vi "View-Scheme.vi"(11 "Material-Scheme.lvclass":refnum<class "Material-Scheme.lvclass">) -> ()   [LabVIEW 2021, in "TSC Material Theme.lvlib" / "Material-Scheme.lvclass"]
doc: "scheme view UI set up like the material theme display\n\n<b>Code Developed By:</b>\nTechnology Service Corporation\nwww.tsc.com/atcs\n\nDeveloper:\nDaniel Coons"
uses:
  Material-Scheme.lvclass
  <vilib>/Utility/traverseref.llb/TRef TravTarget.ctl
  Material-Scheme.lvclass/Material-Scheme.ctl
  <vilib>/Utility/colorconv.llb/Color to RGB.vi
  <vilib>/Utility/traverseref.llb/VI Scripting - Traverse.lvlib
panel:
  out "Scrim":u32(colorbox)
  out "Shadow":u32(colorbox)
  out "Inverse Primary":u32(colorbox)
  out "Inverse on Surface":u32(colorbox)
  out "Inverse Surface":u32(colorbox)
  out "On Error Container":u32(colorbox)
  out "Error Container":u32(colorbox)
  out "On Error":u32(colorbox)
  out "Error":u32(colorbox)
  out "Outline":u32(colorbox)
  out "Outline Variant":u32(colorbox)
  out "On Surface Var":u32(colorbox)
  out "On Surface":u32(colorbox)
  out "Surf Container Highest":u32(colorbox)
  out "Surf Container":u32(colorbox)
  out "Surf Container High":u32(colorbox)
  out "Surf Container Low":u32(colorbox)
  out "Surf Container Lowest":u32(colorbox)
  out "Surface Bright":u32(colorbox)
  out "Surface":u32(colorbox)
  out "Surface Dim":u32(colorbox)
  out "Tertiary Fixed":u32(colorbox)
  out "On Tertiary Fixed Variant":u32(colorbox)
  out "On Tertiary Fixed":u32(colorbox)
  out "Tertiary Fixed Dim":u32(colorbox)
  out "On Tertiary Container":u32(colorbox)
  out "Tertiary Container":u32(colorbox)
  out "On Tertiary":u32(colorbox)
  out "Tertiary":u32(colorbox)
  out "Secondary Fixed":u32(colorbox)
  out "On Secondary Fixed Variant":u32(colorbox)
  out "On Secondary Fixed":u32(colorbox)
  out "Secondary Fixed Dim":u32(colorbox)
  out "On Secondary Container":u32(colorbox)
  out "Secondary Container":u32(colorbox)
  out "On Secondary":u32(colorbox)
  out "Secondary":u32(colorbox)
  out "On Primary Fixed Variant":u32(colorbox)
  out "On Primary Fixed":u32(colorbox)
  out "Primary Fixed Dim":u32(colorbox)
  out "Primary Fixed":u32(colorbox)
  out "On Primary Container":u32(colorbox)
  out "Primary Container":u32(colorbox)
  out "On Primary":u32(colorbox)
  out "Primary":u32(colorbox)
  # "Hover to see color pattern and click to change..."
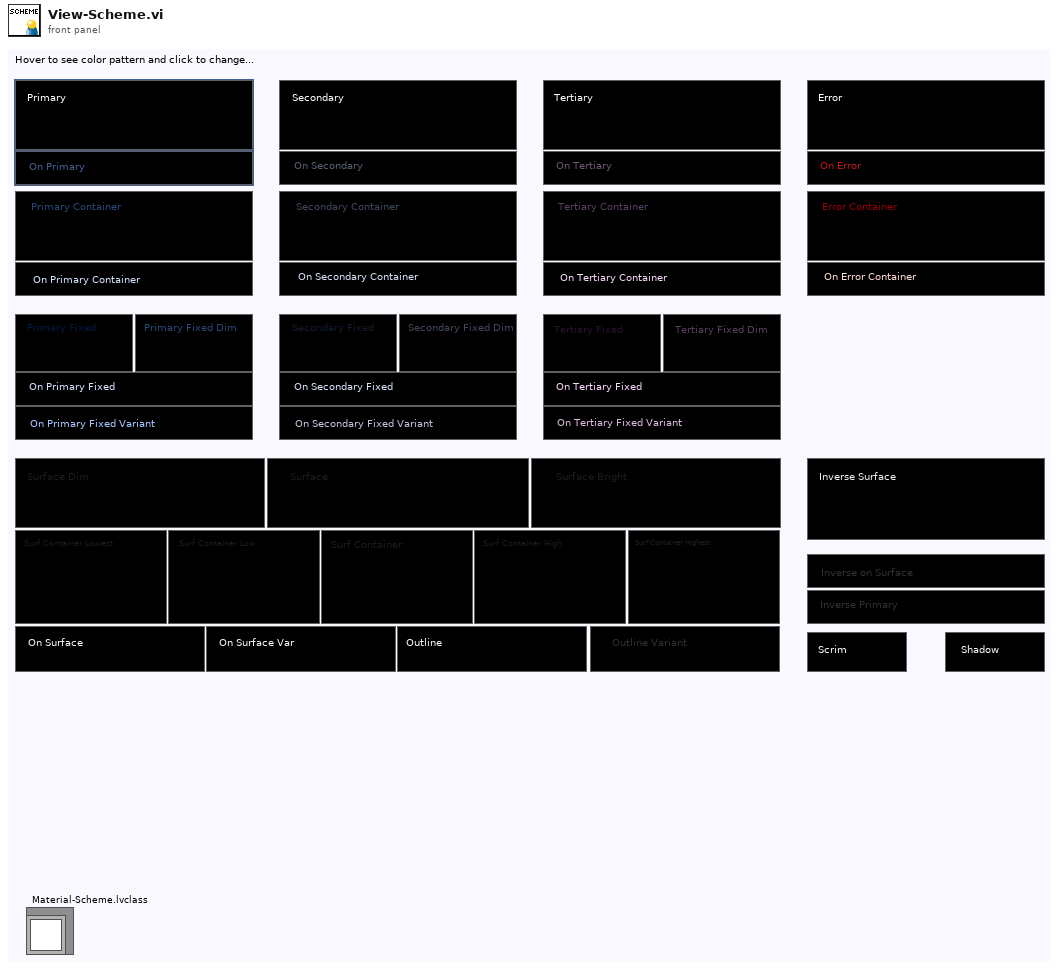
[diagram p1: front panel]
types:
  T1 = typedef "TRef TravTarget.ctl" = enum16{"FP", "BD", "Other"}
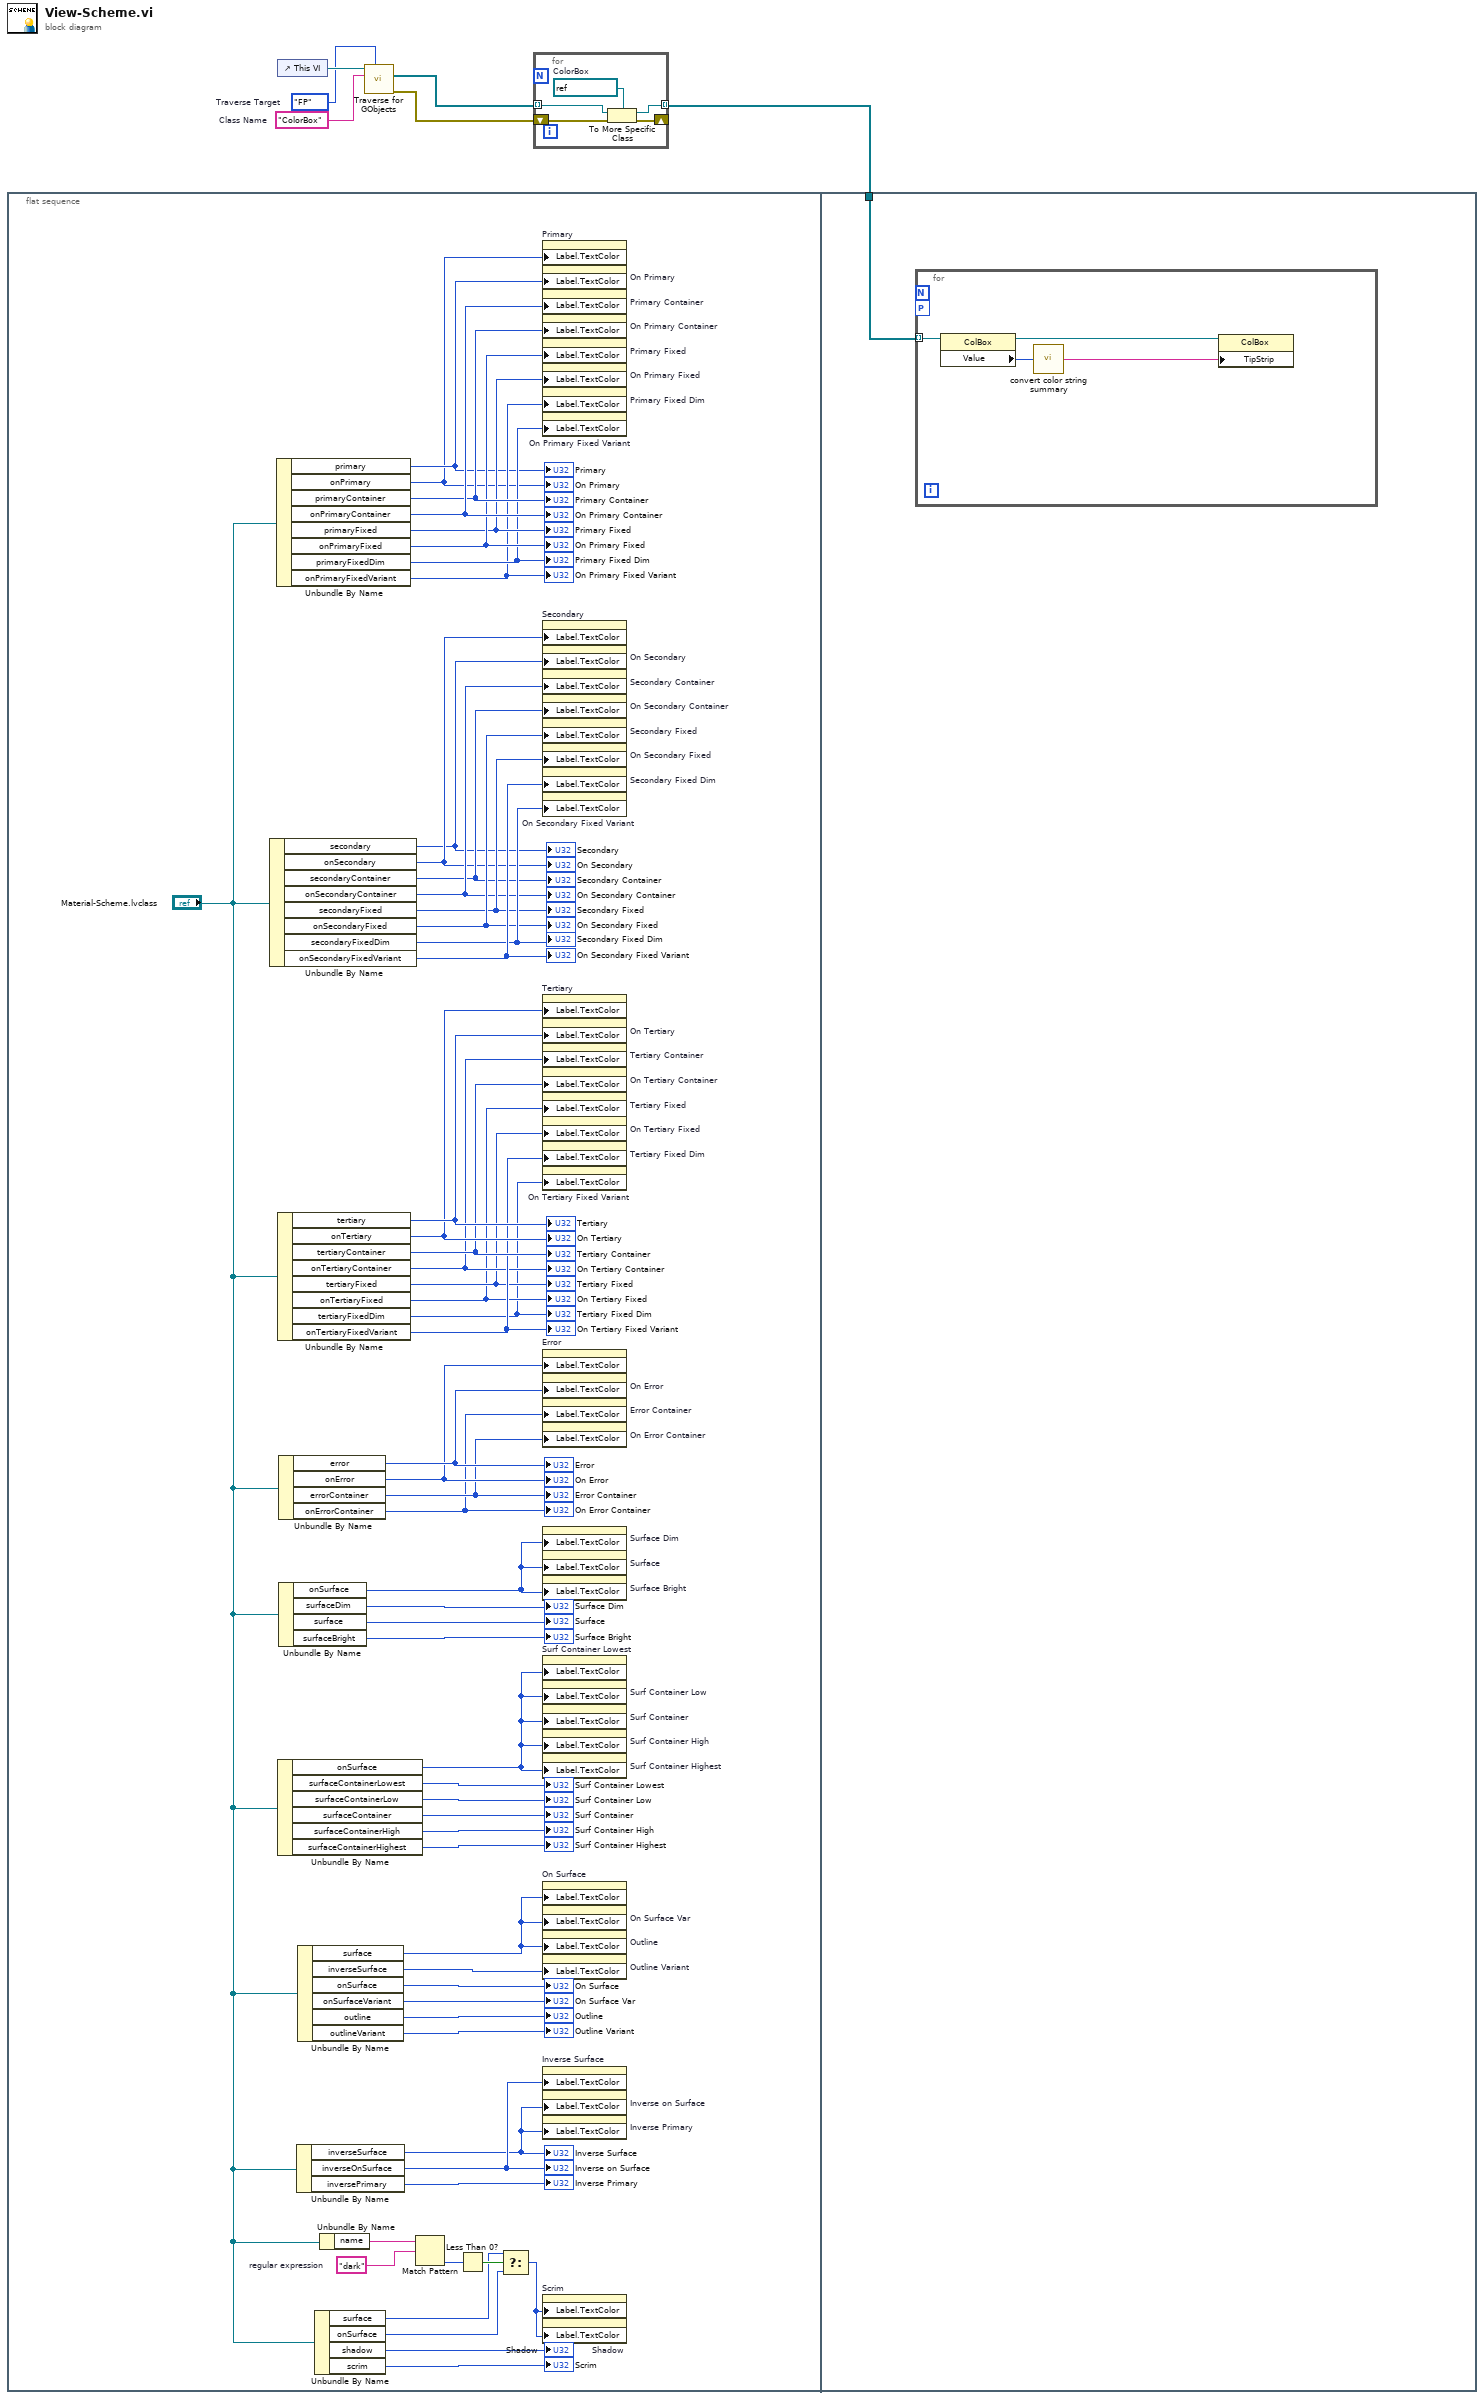
[diagram p0: block diagram]
diagram:
  w3 = TRef_TravTarget."FP"  # Traverse Target
  w6 = "ColorBox"  # Class Name
  n1 = flat-sequence {
    tunnel: w1 -> [w64]
    frame #0 {
      w14 = "dark"  # regular expression
      n2 = Unbundle By Name("Material-Scheme.lvclass") -> ("secondary"=w50:u32, "onSecondary"=w51:u32, "secondaryContainer"=w52:u32, "onSecondaryContainer"=w53:u32, "secondaryFixed"=w54:u32, "onSecondaryFixed"=w55:u32, "secondaryFixedDim"=w56:u32, "onSecondaryFixedVariant"=w57:u32)
      "Secondary" <- w50
      "On Secondary" <- w51
      "Secondary Container" <- w52
      "On Secondary Container" <- w53
      "Secondary Fixed Dim" <- w56
      "On Secondary Fixed" <- w55
      "On Secondary Fixed Variant" <- w57
      "Secondary Fixed" <- w54
      n3 = Unbundle By Name("Material-Scheme.lvclass") -> ("primary"=w8:u32, "onPrimary"=w7:u32, "primaryContainer"=w62:u32, "onPrimaryContainer"=w63:u32, "primaryFixed"=w60:u32, "onPrimaryFixed"=w61:u32, "primaryFixedDim"=w59:u32, "onPrimaryFixedVariant"=w58:u32)
      "Primary" <- w8
      "On Primary" <- w7
      "Primary Container" <- w62
      "On Primary Container" <- w63
      "Primary Fixed" <- w60
      "Primary Fixed Dim" <- w59
      "On Primary Fixed" <- w61
      "On Primary Fixed Variant" <- w58
      n4 = Unbundle By Name("Material-Scheme.lvclass") -> ("tertiary"=w49:u32, "onTertiary"=w48:u32, "tertiaryContainer"=w47:u32, "onTertiaryContainer"=w45:u32, "tertiaryFixed"=w44:u32, "onTertiaryFixed"=w43:u32, "tertiaryFixedDim"=w42:u32, "onTertiaryFixedVariant"=w46:u32)
      "Tertiary" <- w49
      "On Tertiary" <- w48
      "Tertiary Container" <- w47
      "On Tertiary Container" <- w45
      "Tertiary Fixed Dim" <- w42
      "On Tertiary Fixed" <- w43
      "On Tertiary Fixed Variant" <- w46
      "Tertiary Fixed" <- w44
      n5 = Unbundle By Name("Material-Scheme.lvclass") -> ("onSurface"=w28:u32, "surfaceContainerLowest"=→"Surf Container Lowest":u32, "surfaceContainerLow"=→"Surf Container Low":u32, "surfaceContainer"=→"Surf Container":u32, "surfaceContainerHigh"=→"Surf Container High":u32, "surfaceContainerHighest"=→"Surf Container Highest":u32)
      n6 = Unbundle By Name("Material-Scheme.lvclass") -> ("error"=w41:u32, "onError"=w40:u32, "errorContainer"=w39:u32, "onErrorContainer"=w38:u32)
      "Error" <- w41
      "On Error" <- w40
      "Error Container" <- w39
      "On Error Container" <- w38
      n7 = Unbundle By Name("Material-Scheme.lvclass") -> ("onSurface"=w34:u32, "surfaceDim"=→"Surface Dim":u32, "surface"=→"Surface":u32, "surfaceBright"=→"Surface Bright":u32)
      n8 = Unbundle By Name("Material-Scheme.lvclass") -> ("inverseSurface"=w19:u32, "inverseOnSurface"=w20:u32, "inversePrimary"=→"Inverse Primary":u32)
      "Inverse Surface" <- w19
      "Inverse on Surface" <- w20
      n9 = Unbundle By Name("Material-Scheme.lvclass") -> ("surface"=w23:u32, "inverseSurface"=w22:u32, "onSurface"=→"On Surface":u32, "onSurfaceVariant"=→"On Surface Var":u32, "outline"=→"Outline":u32, "outlineVariant"=→"Outline Variant":u32)
      n10 = Unbundle By Name("Material-Scheme.lvclass") -> ("surface"=w11:u32, "onSurface"=w10:u32, "shadow"=→"Shadow":u32, "scrim"=→"Scrim":u32)
      n11 = Unbundle By Name("Material-Scheme.lvclass") -> ("name"=w15:string)
      n12 = Match Pattern(string=w15, regular expression=w14) -> (offset past match=w13:i32)  [unwired: 1 in, 3 out]
      n13 = Less Than 0?(x=w13) -> (x < 0?=w12:bool)
      n14 = Select(t=w11, s=w12, f=w10) -> (s? t:f=w9:u32)
      n15 = property on="Primary" class="ColBox"("Label.TextColor"=w7) -> ()  [unwired: 2 in, 2 out]
      n16 = property on="On Primary" class="ColBox"("Label.TextColor"=w8) -> ()  [unwired: 2 in, 2 out]
      n17 = property on="Primary Container" class="ColBox"("Label.TextColor"=w63) -> ()  [unwired: 2 in, 2 out]
      n18 = property on="On Primary Container" class="ColBox"("Label.TextColor"=w62) -> ()  [unwired: 2 in, 2 out]
      n19 = property on="Primary Fixed" class="ColBox"("Label.TextColor"=w61) -> ()  [unwired: 2 in, 2 out]
      n20 = property on="On Primary Fixed" class="ColBox"("Label.TextColor"=w60) -> ()  [unwired: 2 in, 2 out]
      n21 = property on="Primary Fixed Dim" class="ColBox"("Label.TextColor"=w58) -> ()  [unwired: 2 in, 2 out]
      n22 = property on="On Primary Fixed Variant" class="ColBox"("Label.TextColor"=w59) -> ()  [unwired: 2 in, 2 out]
      n23 = property on="Secondary" class="ColBox"("Label.TextColor"=w51) -> ()  [unwired: 2 in, 2 out]
      n24 = property on="On Secondary" class="ColBox"("Label.TextColor"=w50) -> ()  [unwired: 2 in, 2 out]
      n25 = property on="Secondary Container" class="ColBox"("Label.TextColor"=w53) -> ()  [unwired: 2 in, 2 out]
      n26 = property on="On Secondary Container" class="ColBox"("Label.TextColor"=w52) -> ()  [unwired: 2 in, 2 out]
      n27 = property on="Secondary Fixed" class="ColBox"("Label.TextColor"=w55) -> ()  [unwired: 2 in, 2 out]
      n28 = property on="On Secondary Fixed" class="ColBox"("Label.TextColor"=w54) -> ()  [unwired: 2 in, 2 out]
      n29 = property on="Secondary Fixed Dim" class="ColBox"("Label.TextColor"=w57) -> ()  [unwired: 2 in, 2 out]
      n30 = property on="On Secondary Fixed Variant" class="ColBox"("Label.TextColor"=w56) -> ()  [unwired: 2 in, 2 out]
      n31 = property on="Tertiary" class="ColBox"("Label.TextColor"=w48) -> ()  [unwired: 2 in, 2 out]
      n32 = property on="On Tertiary" class="ColBox"("Label.TextColor"=w49) -> ()  [unwired: 2 in, 2 out]
      n33 = property on="Tertiary Container" class="ColBox"("Label.TextColor"=w45) -> ()  [unwired: 2 in, 2 out]
      n34 = property on="On Tertiary Container" class="ColBox"("Label.TextColor"=w47) -> ()  [unwired: 2 in, 2 out]
      n35 = property on="Tertiary Fixed" class="ColBox"("Label.TextColor"=w43) -> ()  [unwired: 2 in, 2 out]
      n36 = property on="On Tertiary Fixed" class="ColBox"("Label.TextColor"=w44) -> ()  [unwired: 2 in, 2 out]
      n37 = property on="Tertiary Fixed Dim" class="ColBox"("Label.TextColor"=w46) -> ()  [unwired: 2 in, 2 out]
      n38 = property on="On Tertiary Fixed Variant" class="ColBox"("Label.TextColor"=w42) -> ()  [unwired: 2 in, 2 out]
      n39 = property on="Error" class="ColBox"("Label.TextColor"=w40) -> ()  [unwired: 2 in, 2 out]
      n40 = property on="On Error" class="ColBox"("Label.TextColor"=w41) -> ()  [unwired: 2 in, 2 out]
      n41 = property on="Error Container" class="ColBox"("Label.TextColor"=w38) -> ()  [unwired: 2 in, 2 out]
      n42 = property on="On Error Container" class="ColBox"("Label.TextColor"=w39) -> ()  [unwired: 2 in, 2 out]
      n43 = property on="Surface Dim" class="ColBox"("Label.TextColor"=w34) -> ()  [unwired: 2 in, 2 out]
      n44 = property on="Surface" class="ColBox"("Label.TextColor"=w34) -> ()  [unwired: 2 in, 2 out]
      n45 = property on="Surface Bright" class="ColBox"("Label.TextColor"=w34) -> ()  [unwired: 2 in, 2 out]
      n46 = property on="Surf Container Lowest" class="ColBox"("Label.TextColor"=w28) -> ()  [unwired: 2 in, 2 out]
      n47 = property on="Surf Container Low" class="ColBox"("Label.TextColor"=w28) -> ()  [unwired: 2 in, 2 out]
      n48 = property on="Surf Container" class="ColBox"("Label.TextColor"=w28) -> ()  [unwired: 2 in, 2 out]
      n49 = property on="Surf Container High" class="ColBox"("Label.TextColor"=w28) -> ()  [unwired: 2 in, 2 out]
      n50 = property on="Surf Container Highest" class="ColBox"("Label.TextColor"=w28) -> ()  [unwired: 2 in, 2 out]
      n51 = property on="On Surface" class="ColBox"("Label.TextColor"=w23) -> ()  [unwired: 2 in, 2 out]
      n52 = property on="On Surface Var" class="ColBox"("Label.TextColor"=w23) -> ()  [unwired: 2 in, 2 out]
      n53 = property on="Outline" class="ColBox"("Label.TextColor"=w23) -> ()  [unwired: 2 in, 2 out]
      n54 = property on="Outline Variant" class="ColBox"("Label.TextColor"=w22) -> ()  [unwired: 2 in, 2 out]
      n55 = property on="Inverse Surface" class="ColBox"("Label.TextColor"=w20) -> ()  [unwired: 2 in, 2 out]
      n56 = property on="Inverse on Surface" class="ColBox"("Label.TextColor"=w19) -> ()  [unwired: 2 in, 2 out]
      n57 = property on="Inverse Primary" class="ColBox"("Label.TextColor"=w19) -> ()  [unwired: 2 in, 2 out]
      n58 = property on="Scrim" class="ColBox"("Label.TextColor"=w9) -> ()  [unwired: 2 in, 2 out]
      n59 = property on="Shadow" class="ColBox"("Label.TextColor"=w9) -> ()  [unwired: 2 in, 2 out]
    }
    frame #1 {
      n60 = for {
        tunnel: w64 -> [w68] mode=indexing
        workers-P: _ -> [_]
        n61 = property class="ColBox"(reference=w68) -> (reference out=w65:refnum<vi>, "Value"=w66:u32)  [unwired: 1 in, 1 out]
        n62 = call "convert color string summary.vi"("primary"=w66) -> ("String"=w67:string)
        n63 = property on="Property Node" class="ColBox"(reference=w65, "TipStrip"=w67) -> ()  [unwired: 1 in, 2 out]
      }
    }
  }
  n64 = control-ref of="This VI"() -> (w5:refnum<vi>)
  n65 = call <vilib>:"Traverse for GObjects.vi"("Traverse Target"=w3, "Class Name"=w6, "VI Refnum"=w5) -> ("error out"=w2:errorcluster, "References"=w4:refnum<vi>[])  [unwired: 5 in, 2 out]
  n66 = for {
    tunnel: w4 -> [w70] mode=indexing
    shift-right: [w72] -> _
    shift-left: w2 -> [w73]
    tunnel: [w69] -> w1 mode=indexing
    w71 = refnum<vi> refnum  # ColorBox
    n67 = To More Specific Class(target class=w71, reference=w70, error in=w73) -> (specific class reference=w69:refnum<vi>, error out=w72:errorcluster)
  }
